vi "Read Device Dependent Error.vi"(8 "error in (no error)":errorcluster, 11 "VISA resource name":refnum<visa-resource-name>) -> (0 "error out":errorcluster, 1 "Error Message":string, 2 "Error Code":i32, 3 "VISA resource name out":refnum<visa-resource-name>)   [LabVIEW 2013, in "LeCroy Wave Series.lvlib"]
doc: "Reads and clears the contents of the Device Dependent or device specific error Register (DDR). In the case of a hardware failure, the DDR register specifies the origin of the failure."
uses:
  LeCroy Wave Series.lvlib
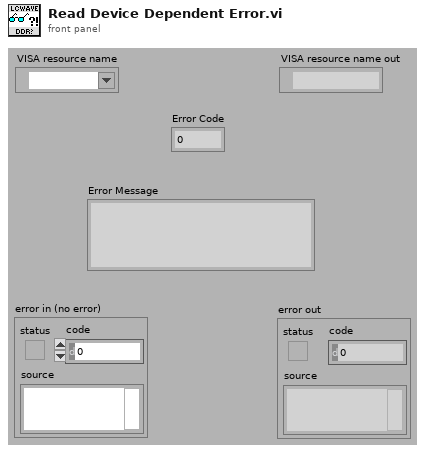
[diagram p1: front panel]
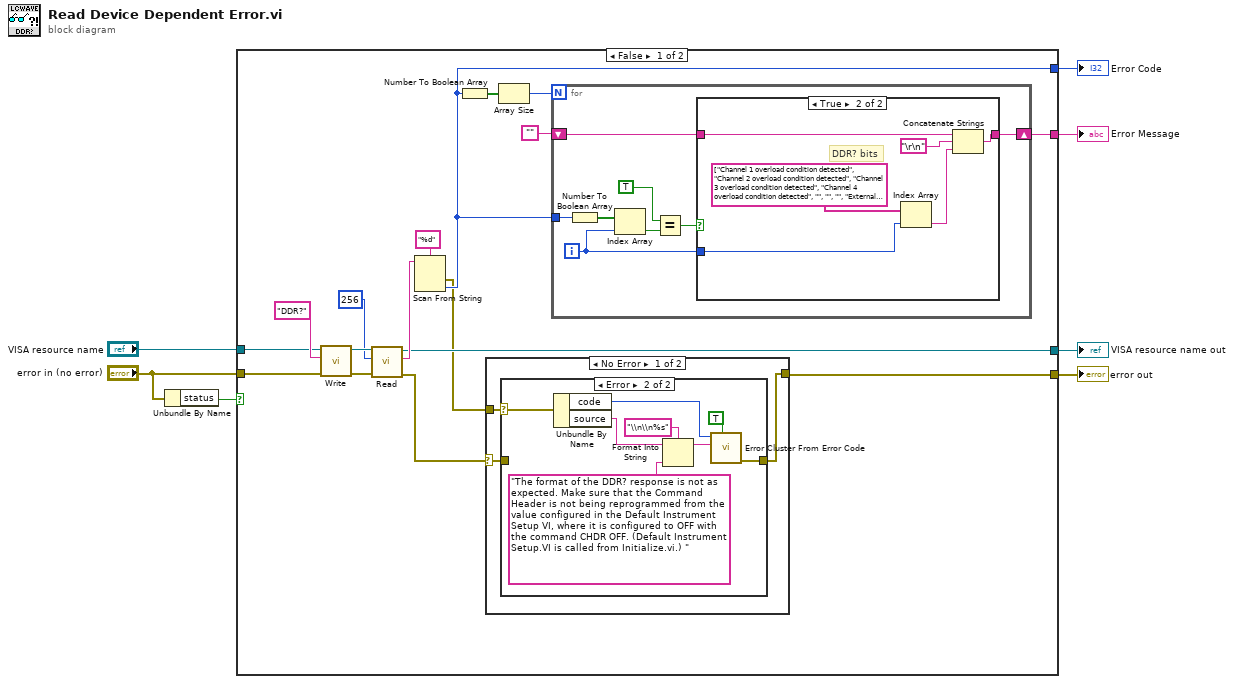
[diagram p0: block diagram]
diagram:
  n1 = Unbundle By Name("error in (no error)") -> ("status"=w1:bool)
  n2 = case shown="False" w1 {
    tunnel: [w16 _] -> w7
    tunnel: "VISA resource name" -> [w15 w54]
    tunnel: "error in (no error)" -> [w14 w53]
    tunnel: [w13 w54] -> w5
    tunnel: [w8 w53] -> w4
    tunnel: [w11 _] -> w3
    frame False {
      n3 = call "Write.vi"("error in (no error)"=w14, "Write Buffer"="DDR?" ("write buffer"), "VISA resource name"=w15) -> ("error out"=w23:errorcluster, "VISA resource name out"=w24:refnum<visa-resource-name>)  [unwired: 6 in, 1 out]
      n4 = call "Read.vi"("error in (no error)"=w23, "Byte Count"=u32 256 ("byte count"), "VISA resource name"=w24) -> ("error out"=w9:errorcluster, "Read Buffer"=w20:string, "VISA resource name out"=w13:refnum<visa-resource-name>)  [unwired: 5 in, 1 out]
      n5 = Scan From String(format string="%d", input string=w20) -> (error out=w10:errorcluster, output 1=w16:i32)  [unwired: 3 in, 2 out]
      n6 = Number To Boolean Array(number=w16) -> (Boolean array=w18:bool[])
      n7 = case shown="No Error" w9 {
        selector: w9 -> [w27 w37]
        tunnel: [w26 w37] -> w8
        tunnel: w10 -> [w25 _]
        frame No Error {
          n8 = case shown="Error" w25 {
            selector: w25 -> [_ w32]
            tunnel: w27 -> [w28 _]
            tunnel: [w28 w35] -> w26
            frame No Error {
            }
            frame Error {
              n9 = Unbundle By Name(w32) -> ("code"=w31:i32, "source"=w30:string)
              n10 = Format Into String(format string="\\n\\n%s", initial string=w30, "The format of the DDR? response is not as expected. Make sure that the Command Header is not being reprogrammed from the value configured in the Default Instrument Setup VI, where it is configured to OFF with the command CHDR OFF. (Default Instrument Setup.VI is called from Initialize.vi.) " ("source")) -> (resulting string=w29:string)  [unwired: 1 in, 1 out]
              n11 = call <vilib>:"Error Cluster From Error Code.vi"("show call chain? (False)"=TRUE, "error message (\"\")"=w29, "error code (0)"=w31) -> ("error out"=w35:errorcluster)  [unwired: 6 in]
            }
          }
        }
        frame Error {
        }
      }
      n12 = Array Size(array=w18) -> (size(s)=w17:i32)
      n13 = for {
        N: w17 -> [_]
        tunnel: w16 -> [w45]
        shift-right: [w39] -> w11
        shift-left: "" ("Empty String Constant") -> [w40]
        i -> [w38]
        n14 = Number To Boolean Array(number=w45) -> (Boolean array=w44:bool[])
        n15 = Index Array(array=w44, index=w38) -> (element=w43:bool)
        n16 = Equal?(x=TRUE, y=w43) -> (x = y?=w41:bool)
        n17 = case shown="True" w41 {
          tunnel: w40 -> [w46 w52]
          tunnel: [w46 w50] -> w39
          tunnel: w38 -> [_ w48]
          frame False {
          }
          frame True {
            # "DDR? bits"
            n18 = Index Array(array=string[] ["Channel 1 overload condition detected", "Channel 2 overload condition detected", "Channel 3 overload condition detected", "Channel 4 overload condition detected", "", "", "", "External input overload condition detected", "Channel 1 hardware failure detected", "Channel 2 hardware failure detected", "Channel 3 hardware failure detected", "Channel 4 hardware failure detected", "Trigger hardware failure detected", "Timebase hardware failure detected"], index=w48) -> (element=w47:string)
            n19 = Concatenate Strings(w52, "\r\n" ("End of Line Constant"), w47) -> (w50:string)
          }
        }
      }
    }
    frame True {
    }
  }
  "VISA resource name out" <- w5
  "error out" <- w4
  "Error Message" <- w3
  "Error Code" <- w7
